vi "Get_temporary_save_path_171213.vi"(3 "Temporary file name prefix":string="TrackTemp") -> (0 "Temporary file output path":path, 1 "date/time string":string)   [LabVIEW 2016]
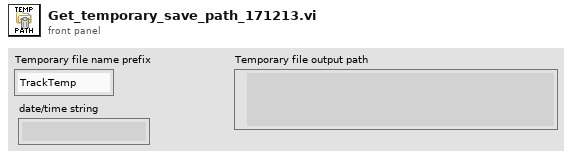
[diagram p1: front panel]
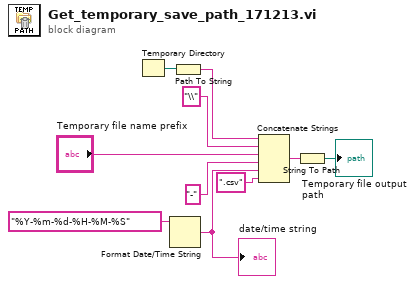
[diagram p0: block diagram]
diagram:
  n1 = Temporary Directory() -> (w8:path)
  n2 = Format Date/Time String(time format string (%c)="%Y-%m-%d-%H-%M-%S") -> (date/time string=w1:string)  [unwired: 2 in]
  "date/time string" <- w1
  n3 = Path To String(path=w8) -> (string=w7:string)
  n4 = Concatenate Strings(w7, "\\" ("string"), "Temporary file name prefix", "-" ("string"), w1, ".csv" ("string")) -> (w10:string)
  n5 = String To Path(string=w10) -> (path=→"Temporary file output path":path)
